vi "UpgradeFirmware.vi"(8 "error in (no error)":errorcluster, 9 "DevInfo":T3={"Hostname"="", "IPAddress"="", "MAC"="", "SerialNum"="", "Model"="", "Status"="", "FW"="", "OSDesc"="", "ImgTitle"="", "ImgDesc"="", "ImgVer"="", "ImgID"="", "IP Address Request Mode"=1, "SubnetMask"="", "Gateway"="", "DNSServer"=""} {"IP Address Request Mode" items=["Static"=1, "DHCP/Link-Local"=2, "Link-Local Only"=4, "DHCP Only"=8]}, 10 "AppImage Properties":T1, 11 "Selected Image File":path) -> (0 "error out":errorcluster)   [LabVIEW 2021]
uses:
  TypeDefs/DevInfo.ctl
  TypeDefs/AppImageProperties.ctl
  TypeDefs/FPGA_Properties_Element.ctl
  TypeDefs/TargetAccess.ctl
  <vilib>/nisyscfg/Upgrade Firmware (File).vi
  <vilib>/nisyscfg/Close (System).vi
  <vilib>/nisyscfg/nisyscfg.lvlib
  <resource>/objmgr/nisysapi.rc
panel:
  in  "Stop Checking for Events":bool
  out "Progress":i8(slide) scale=0.0..100.0
  out "Status":string
  # "Upgrading Firmware"
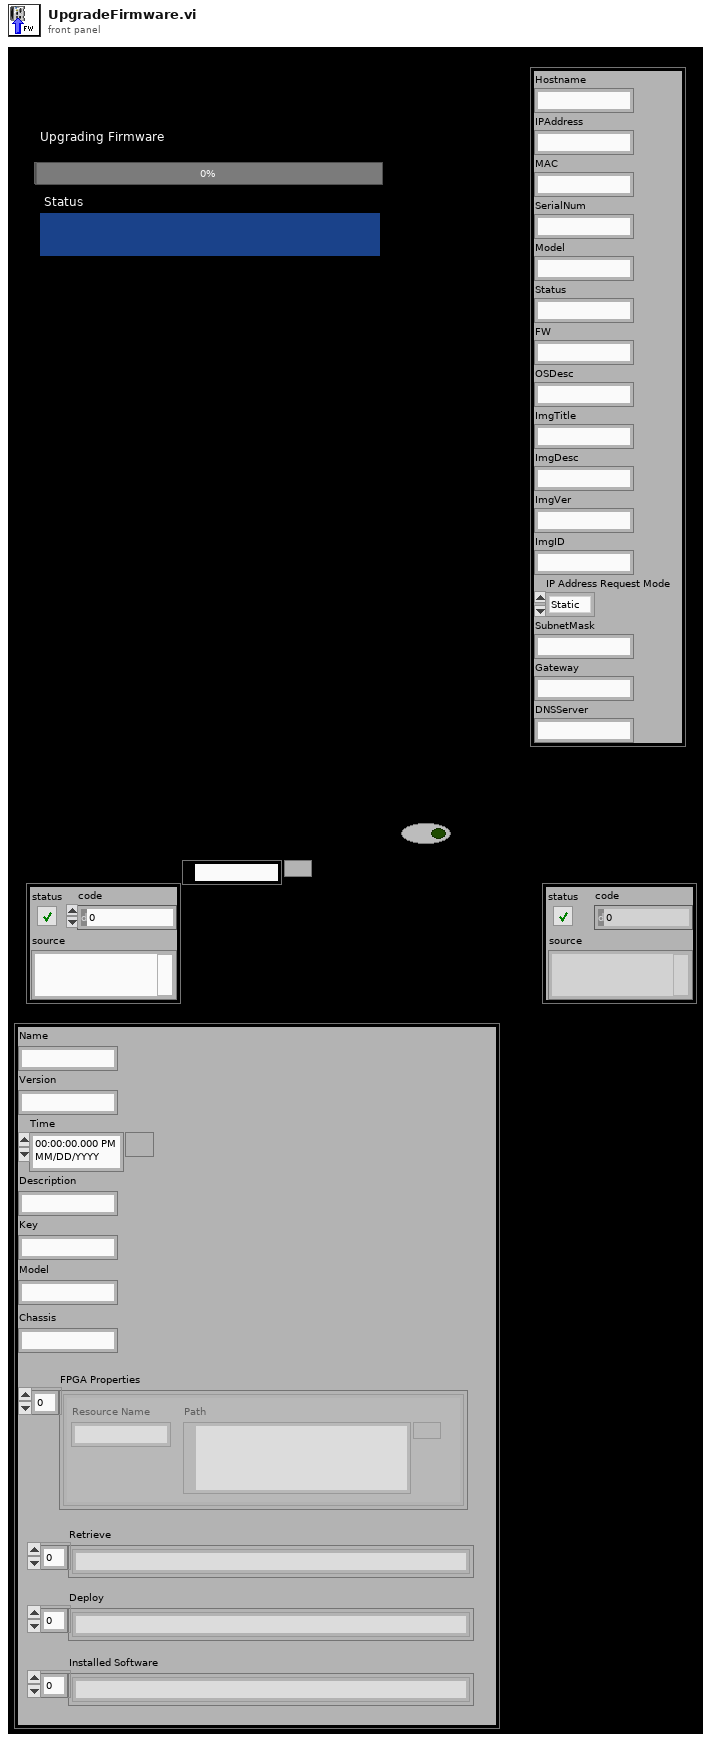
[diagram p1: front panel]
types:
  T1 = typedef "AppImageProperties.ctl" = cluster{"Name":string, "Version":string, "Time":timestamp, "Description":string, "Key":string, "Chassis":string, "FPGA Properties":T2[], "Model":string, "Retrieve":string[], "Deploy":string[], "Installed Software":string[]}
  T2 = typedef "FPGA_Properties_Element.ctl" = cluster{"Resource Name":string, "Path":path}
  T3 = typedef "DevInfo.ctl" = cluster{"Hostname":string, "IPAddress":string, "MAC":string, "SerialNum":string, "Model":string, "Status":string, "FW":string, "OSDesc":string, "ImgTitle":string, "ImgDesc":string, "ImgVer":string, "ImgID":string, "IP Address Request Mode":i32, "SubnetMask":string, "Gateway":string, "DNSServer":string}
  T4 = typedef "TargetAccess.ctl" = enum16{"Read-Only", "Admin"}
  T5 = enum32{"state changed", "beginning restart", "getting file", "putting file", "creating directory", "deleting file", "deleting directory", "enumerating file system", "renaming file", "current component", "operation progress", "downloading file", "unpacking file", "running install script", "creating image", "validating image", "applying image", "beginning format", "completing format"}
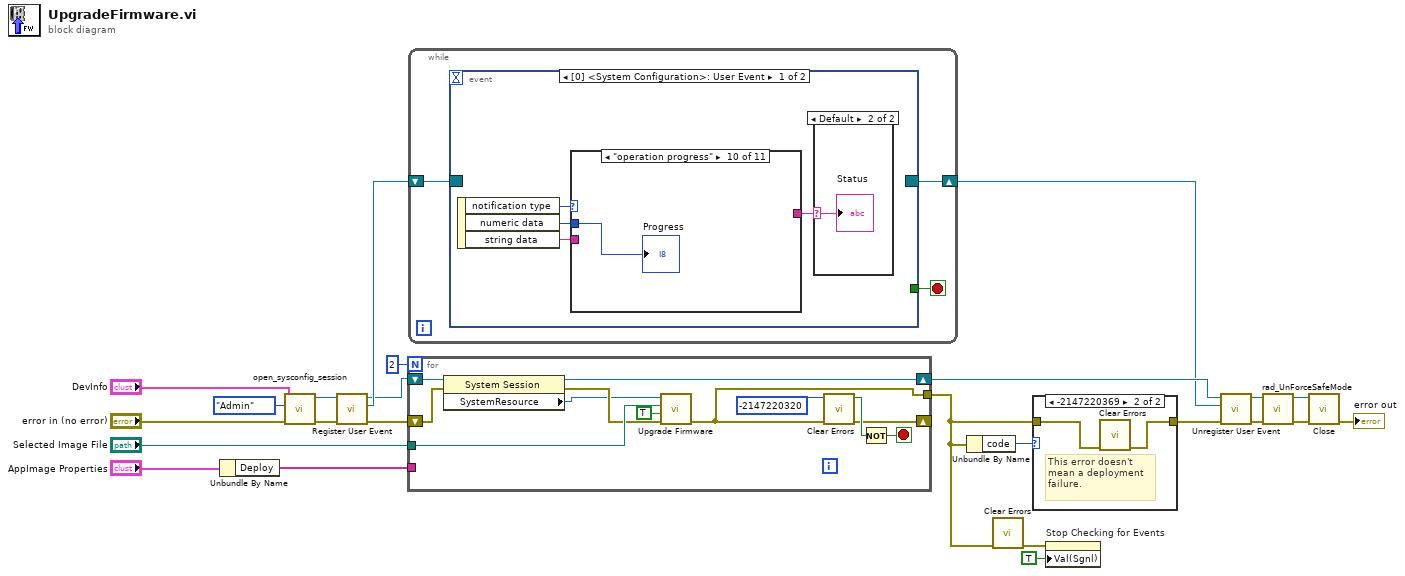
[diagram p0: block diagram]
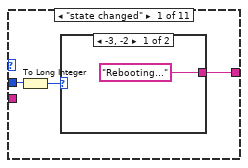
[diagram p4: hidden frame]
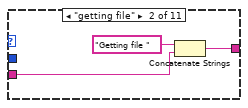
[diagram p6: hidden frame]
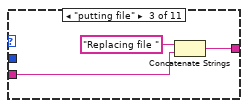
[diagram p7: hidden frame]
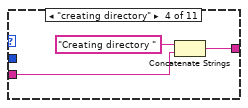
[diagram p8: hidden frame]
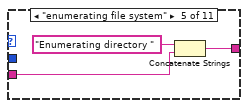
[diagram p9: hidden frame]
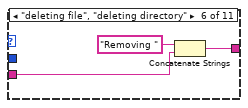
[diagram p10: hidden frame]
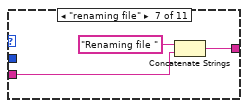
[diagram p11: hidden frame]
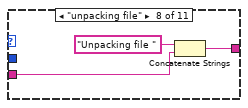
[diagram p12: hidden frame]
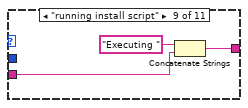
[diagram p13: hidden frame]
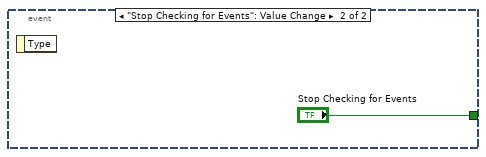
[diagram p15: hidden frame]
diagram:
  n1 = Unbundle By Name("AppImage Properties") -> ("Deploy"=w18:string[])
  n2 = call "open_sysconfig_session.vi"("error in (no error)"="error in (no error)", "Target Access"=TargetAccess."Admin", "DevInfo"="DevInfo") -> ("error out"=w22:errorcluster, "Session Out"=w21:refnum<k21>)  [unwired: 6 in, 1 out]
  n3 = call <vilib>:"Register User Event.vi"("error in (no error)"=w22, "Session in"=w21) -> ("error out"=w13:errorcluster, "Event Registration out"=w15:refnum<event-registration>, "Session out"=w1:refnum<k21>)  [unwired: 7 in]
  n4 = for {
    N: 2 -> [_]
    tunnel: "Selected Image File" -> [w32]
    tunnel: w18 -> [_]
    tunnel: [w31] -> w11
    shift-right: [w34] -> _
    shift-left: w13 -> [w28]
    shift-right: [w29] -> w8
    shift-left: w1 -> [w30]
    stop <- w36 stop-if-true
    n5 = property class="System Session"(reference=w30, error in=w28) -> (reference out=w29:refnum<k21>, error out=w27:errorcluster, "SystemResource"=w26:refnum<k20>)
    n6 = call-poly <vilib>:"Upgrade Firmware.vi"("error in (no error)"=w27, "Always Overwrite (F)"=TRUE, "Firmware File"=w32, "Resource in"=w26) -> ("error out"=w31:errorcluster)  [unwired: 4 in, 3 out]
    n7 = call <vilib>:"Clear Errors.vi"("error in (no error)"=w31, "specific error code to clear (0: all)"=-2147220320) -> ("error out"=w34:errorcluster, "specific error cleared?"=w35:bool)  [unwired: 4 in]
    n8 = Not(x=w35) -> (.not. x?=w36:bool)
  }
  n9 = while {
    shift-right: [w37] -> w7
    shift-left: w15 -> [w39]
    stop <- w38 stop-if-true
    n10 = event shown="[0] <System Configuration>: User Event" {
      selector: w39 -> [_ _]
      dyn-events: [_ _] -> w37
      timeout: _ -> [_ _]
      tunnel: [_ "Stop Checking for Events"] -> w38
      event User Event {
        n11 = event-data() -> ("notification type"=w43:T5, "numeric data"=w41:u32, "string data"=w42:string)  [unwired: 1 in]
        n12 = case shown="\"operation progress\"" w43 {
          tunnel: [w45 w49 w52 w55 w58 w61 w64 w67 w70 _ _] -> w40
          tunnel: w42 -> [_ w50 w53 w56 w59 w62 w65 w68 w71 _ _]
          tunnel: w41 -> [w47 _ _ _ _ _ _ _ _ w73 _]
          frame "state changed" {
            n13 = To Long Integer(number=w47) -> (32bit integer=w46:i32)
            n14 = case shown="-3, -2" w46 {
              tunnel: ["Rebooting..." _] -> w45
              frame -3, -2 {
              }
              frame Default {
              }
            }
          }
          frame "getting file" {
            n15 = Concatenate Strings("Getting file " ("Status"), w50) -> (w49:string)
          }
          frame "putting file" {
            n16 = Concatenate Strings("Replacing file " ("Status"), w53) -> (w52:string)
          }
          frame "creating directory" {
            n17 = Concatenate Strings("Creating directory " ("Status"), w56) -> (w55:string)
          }
          frame "enumerating file system" {
            n18 = Concatenate Strings("Enumerating directory " ("Status"), w59) -> (w58:string)
          }
          frame "deleting file", "deleting directory" {
            n19 = Concatenate Strings("Removing " ("Status"), w62) -> (w61:string)
          }
          frame "renaming file" {
            n20 = Concatenate Strings("Renaming file " ("Status"), w65) -> (w64:string)
          }
          frame "unpacking file" {
            n21 = Concatenate Strings("Unpacking file " ("Status"), w68) -> (w67:string)
          }
          frame "running install script" {
            n22 = Concatenate Strings("Executing " ("Status"), w71) -> (w70:string)
          }
          frame "operation progress" {
            "Progress" <- w73
          }
          frame Default {
          }
        }
        n23 = case shown="Default" w40 {
          selector: w40 -> [_ w44]
          frame "" {
          }
          frame Default {
            "Status" <- w44
          }
        }
      }
      event "Stop Checking for Events": Value Change {
        n24 = event-data() -> ()  [unwired: 1 in, 1 out]
      }
    }
  }
  n25 = Unbundle By Name(w11) -> ("code"=w12:i32)
  n26 = call <vilib>:"Clear Errors.vi"("error in (no error)"=w11) -> ("error out"=w10:errorcluster)  [unwired: 5 in, 1 out]
  n27 = case shown="-2147220369" w12 {
    tunnel: w11 -> [w75 w77]
    tunnel: [w75 w76] -> w9
    frame Default {
    }
    frame -2147220369 {
      # "This error doesn't\nmean a deployment\nfailure."
      n28 = call <vilib>:"Clear Errors.vi"("error in (no error)"=w77) -> ("error out"=w76:errorcluster)  [unwired: 5 in, 1 out]
    }
  }
  n29 = property on="Stop Checking for Events" class="Bool (strict)"(error in=w10, "Val(Sgnl)"=TRUE ("Value (Signaling)")) -> ()  [unwired: 1 in, 2 out]
  n30 = call <vilib>:"Unregister User Event.vi"("error in (no error)"=w9, "Event Registration in"=w7, "Session in"=w8) -> ("error out"=w5:errorcluster, "Session out"=w6:refnum<k21>)  [unwired: 7 in]
  n31 = call "rad_UnForceSafeMode.vi"("error in (no error)"=w5, "Target in"=w6) -> ("error out"=w3:errorcluster, "Target out"=w4:refnum<k21>)  [unwired: 8 in]
  n32 = call-poly <vilib>:"Close.vi"("error in (no error)"=w3, "Session in"=w4) -> ("error out"=→"error out":errorcluster)  [unwired: 9 in]
